vi "SRSLA.vi"(8 "error in (no error)":errorcluster, 11 "VISA resource name":refnum<visa-resource-name>="GPIB2::13::INSTR") -> (0 "error out":errorcluster, 1 "Theta":dbl, 2 "X":dbl, 3 "VISA resource name out":refnum<visa-resource-name>, 4 "Y":dbl, 5 "Data_cluster":dbl[](array[numeric]), 6 "R":dbl, 7 "Aux in 1":dbl, 9 "Aux in 2":dbl)   [LabVIEW 2023]
uses:
  Program Files/National Instruments/LabVIEW 2023/instr.lib/Stanford Research 830/Public/Data/Read (1 Parameter).vi
  Program Files/National Instruments/LabVIEW 2023/instr.lib/Stanford Research 830/Stanford Research 830.lvlib
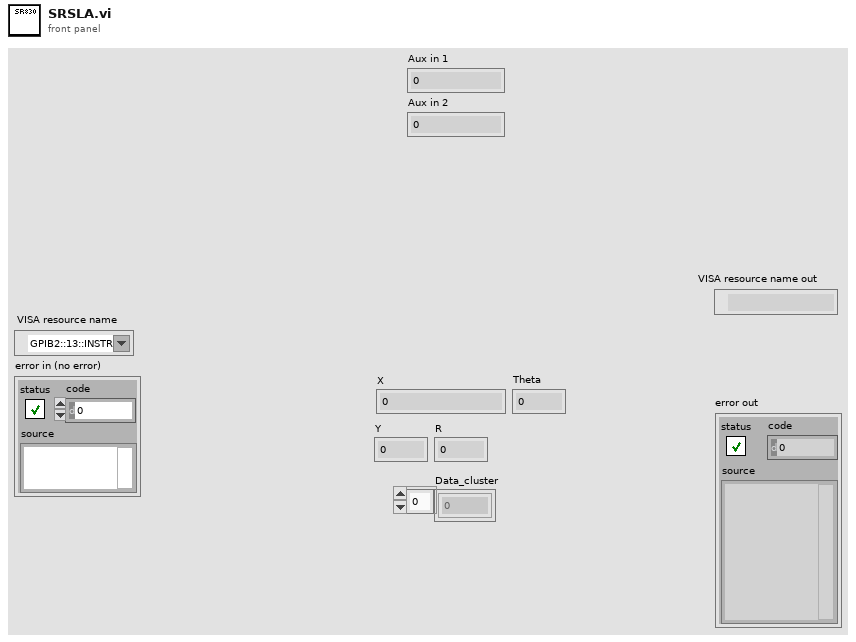
[diagram p1: front panel]
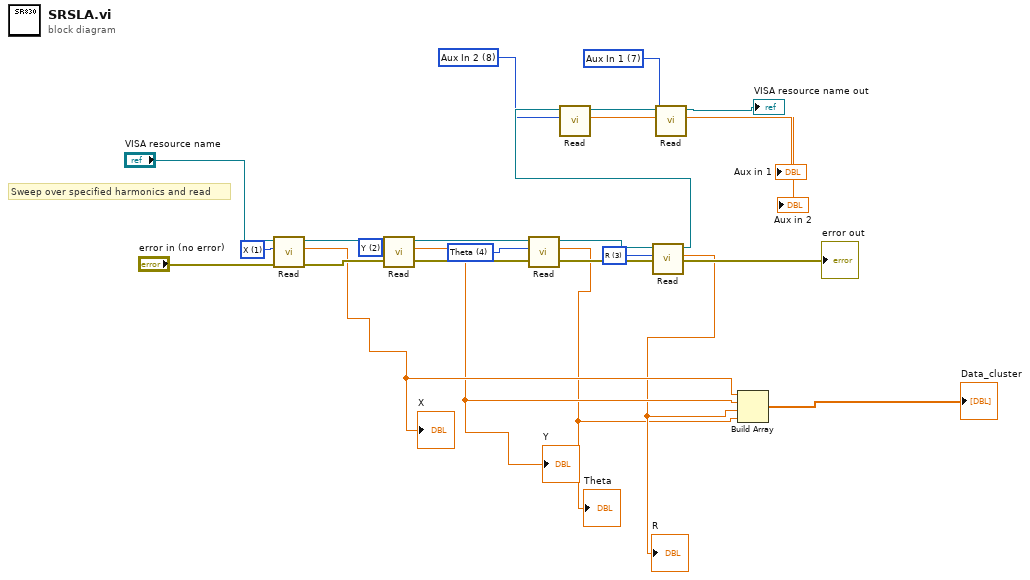
[diagram p0: block diagram]
diagram:
  w3 = u16 8 items=["X"=1, "Y"=2, "R"=3, "Theta"=4, "Channel 1"=5, "Channel 2"=6, "Aux In 1"=7, "Aux In 2"=8, "Aux In 3"=9, "Aux In 4"=10] ("Parameter (1: X)")
  w4 = u16 7 items=["X"=1, "Y"=2, "R"=3, "Theta"=4, "Channel 1"=5, "Channel 2"=6, "Aux In 1"=7, "Aux In 2"=8, "Aux In 3"=9, "Aux In 4"=10] ("Parameter (1: X)")
  w13 = u16 3 items=["X"=1, "Y"=2, "R"=3, "Theta"=4, "Channel 1"=5, "Channel 2"=6, "Aux In 1"=7, "Aux In 2"=8, "Aux In 3"=9, "Aux In 4"=10] ("Parameter (1: X)")
  w15 = u16 4 items=["X"=1, "Y"=2, "R"=3, "Theta"=4, "Channel 1"=5, "Channel 2"=6, "Aux In 1"=7, "Aux In 2"=8, "Aux In 3"=9, "Aux In 4"=10] ("Parameter (1: X)")
  w17 = u16 2 items=["X"=1, "Y"=2, "R"=3, "Theta"=4, "Channel 1"=5, "Channel 2"=6, "Aux In 1"=7, "Aux In 2"=8, "Aux In 3"=9, "Aux In 4"=10] ("Parameter (1: X)")
  w19 = u16 1 items=["X"=1, "Y"=2, "R"=3, "Theta"=4, "Channel 1"=5, "Channel 2"=6, "Aux In 1"=7, "Aux In 2"=8, "Aux In 3"=9, "Aux In 4"=10] ("Parameter (1: X)")
  # "Sweep over specified harmonics and read"
  n1 = call-poly "Read.vi"("error in (no error)"="error in (no error)", "Parameter (1: X)"=w19, "VISA resource name"="VISA resource name") -> ("error out"=→"error out":errorcluster, "Measurement"=w12:dbl, "VISA resource name out"=w18:refnum<visa-resource-name>)  [unwired: 6 in]
  "X" <- w12
  n2 = call-poly "Read.vi"("Parameter (1: X)"=w17, "VISA resource name"=w18) -> ("Measurement"=w11:dbl, "VISA resource name out"=w16:refnum<visa-resource-name>)  [unwired: 7 in, 1 out]
  "Y" <- w11
  n3 = call-poly "Read.vi"("Parameter (1: X)"=w15, "VISA resource name"=w16) -> ("Measurement"=w9:dbl, "VISA resource name out"=w14:refnum<visa-resource-name>)  [unwired: 7 in, 1 out]
  "Theta" <- w9
  n4 = call-poly "Read.vi"("Parameter (1: X)"=w13, "VISA resource name"=w14) -> ("Measurement"=w10:dbl, "VISA resource name out"=w7:refnum<visa-resource-name>)  [unwired: 7 in, 1 out]
  "R" <- w10
  n5 = call-poly "Read.vi"("Parameter (1: X)"=w3, "VISA resource name"=w7) -> ("Measurement"=→"Aux in 2":dbl, "VISA resource name out"=w6:refnum<visa-resource-name>)  [unwired: 7 in, 1 out]
  n6 = call-poly "Read.vi"("Parameter (1: X)"=w4, "VISA resource name"=w6) -> ("Measurement"=→"Aux in 1":dbl, "VISA resource name out"=→"VISA resource name out":refnum<visa-resource-name>)  [unwired: 7 in, 1 out]
  n7 = Build Array(w12, w11, w10, w9) -> (→"Data_cluster":dbl[])
